vi "Write Run_.vi"(8 "error in (no error)":errorcluster, 10 "Run?":bool, 11 "CnPt in":refnum<class "CnPt.lvclass">) -> (0 "error out":errorcluster, 3 "CnPt out":refnum<class "CnPt.lvclass">)   [LabVIEW 2015, in "CnPt.lvclass"]
uses:
  CnPt.lvclass
  CnPt.lvclass/CnPt.ctl
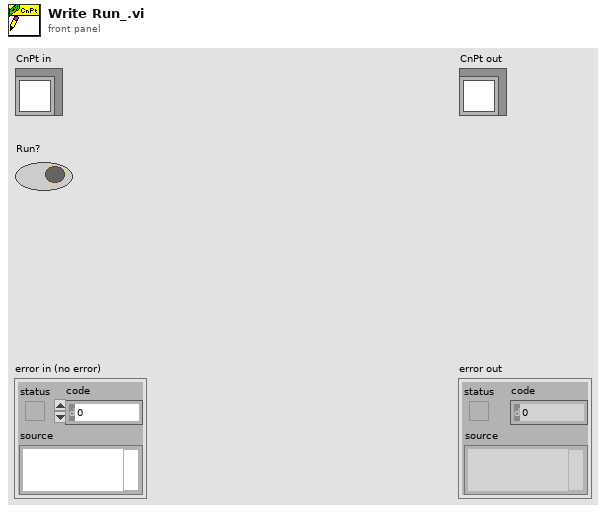
[diagram p1: front panel]
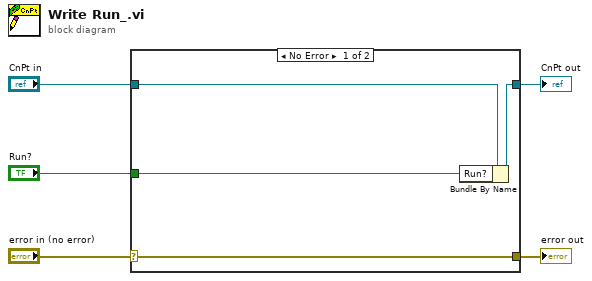
[diagram p0: block diagram]
diagram:
  n1 = case shown="No Error" "error in (no error)" {
    selector: "error in (no error)" -> [w9 w10]
    tunnel: [w9 w10] -> w4
    tunnel: [w7 w11] -> w2
    tunnel: "CnPt in" -> [w8 w11]
    tunnel: "Run?" -> [w6 _]
    frame No Error {
      n2 = Bundle By Name(cluster=w8, "Run?"=w6) -> (w7:refnum<class "CnPt.lvclass">)
    }
    frame Error {
    }
  }
  "error out" <- w4
  "CnPt out" <- w2
